vi "OAT Tachless Keep Plot Scale Range Consistent.vi"(7 "XY Max Range":T1 {"YScale.Range"."Start" format="%.2f"; "YScale.Range"."Minor Incr" format="%.2f"; "YScale.Range"."Increment" format="%.2f"; "YScale.Range"."Maximum" format="%.2f"; "YScale.Range"."Minimum" format="%.2f"; "XScale.Range"."Start" format="%.2f"; "XScale.Range"."Minor Incr" format="%.2f"; "XScale.Range"."Increment" format="%.2f"; "XScale.Range"."Maximum" format="%.2f"; "XScale.Range"."Minimum" format="%.2f"}, 9 "Wavefor Plot ref":refnum<vi>, 10 "TF Plot Ref":refnum<vi>, 11 "Tracks Ref":refnum<vi>) -> ()   [LabVIEW 2017, in "SoundVib_Tachless.lvlib"]
uses:
  <vilib>/addons/Sound and Vibration/Order Analysis/Tachless/SoundVib_Tachless.lvlib
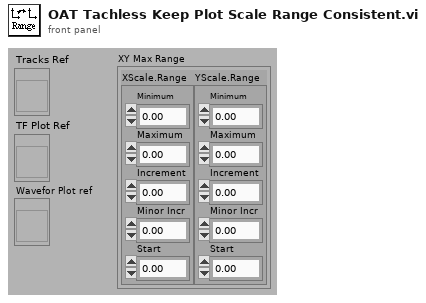
[diagram p1: front panel]
types:
  T1 = cluster{"XScale.Range":cluster{"Minimum":dbl, "Maximum":dbl, "Increment":dbl, "Minor Incr":dbl, "Start":dbl}, "YScale.Range":cluster{"Minimum":dbl, "Maximum":dbl, "Increment":dbl, "Minor Incr":dbl, "Start":dbl}}
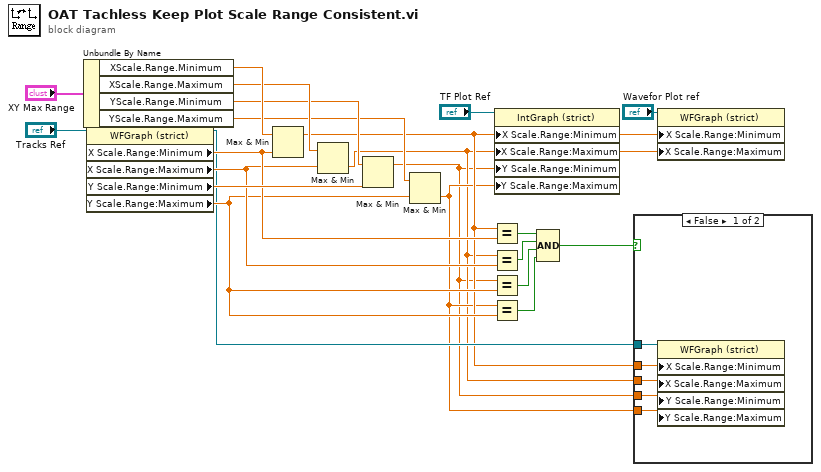
[diagram p0: block diagram]
diagram:
  n1 = Unbundle By Name("XY Max Range") -> ("XScale.Range.Minimum"=w18:dbl, "XScale.Range.Maximum"=w17:dbl, "YScale.Range.Minimum"=w15:dbl, "YScale.Range.Maximum"=w14:dbl)
  n2 = property on="Property Node" class="WFGraph (strict)"(reference="Tracks Ref") -> (reference out=w5:refnum<vi>, "X Scale.Range:Minimum"=w13:dbl, "X Scale.Range:Maximum"=w12:dbl, "Y Scale.Range:Minimum"=w16:dbl, "Y Scale.Range:Maximum"=w11:dbl)  [unwired: 1 in, 1 out]
  n3 = Max & Min(x=w18, y=w13) -> (max(x,y)=w4:dbl)  [unwired: 1 out]
  n4 = Max & Min(x=w17, y=w12) -> (min(x,y)=w2:dbl)  [unwired: 1 out]
  n5 = Max & Min(x=w15, y=w16) -> (max(x,y)=w1:dbl)  [unwired: 1 out]
  n6 = Max & Min(x=w14, y=w11) -> (min(x,y)=w3:dbl)  [unwired: 1 out]
  n7 = Equal?(x=w4, y=w13) -> (x = y?=w10:bool)
  n8 = Equal?(x=w2, y=w12) -> (x = y?=w9:bool)
  n9 = Equal?(x=w1, y=w11) -> (x = y?=w8:bool)
  n10 = Equal?(x=w3, y=w11) -> (x = y?=w7:bool)
  n11 = property on="Property Node" class="IntGraph (strict)"(reference="TF Plot Ref", "X Scale.Range:Minimum"=w4, "X Scale.Range:Maximum"=w2, "Y Scale.Range:Minimum"=w1, "Y Scale.Range:Maximum"=w3) -> ()  [unwired: 1 in, 2 out]
  n12 = Compound Arithmetic op=AND(w10, w9, w8, w7) -> (w6:bool)
  n13 = case shown="False" w6 {
    tunnel: w5 -> [w27 _]
    tunnel: w4 -> [w26 _]
    tunnel: w2 -> [w25 _]
    tunnel: w1 -> [w24 _]
    tunnel: w3 -> [w23 _]
    frame False {
      n14 = property on="Property Node" class="WFGraph (strict)"(reference=w27, "X Scale.Range:Minimum"=w26, "X Scale.Range:Maximum"=w25, "Y Scale.Range:Minimum"=w24, "Y Scale.Range:Maximum"=w23) -> ()  [unwired: 1 in, 2 out]
    }
    frame True {
    }
  }
  n15 = property on="Property Node" class="WFGraph (strict)"(reference="Wavefor Plot ref", "X Scale.Range:Minimum"=w4, "X Scale.Range:Maximum"=w2) -> ()  [unwired: 1 in, 2 out]
